vi "Read.vi"(8 "error in (no error)":errorcluster, 11 "I32 Array in":refnum<class "I32 Array.lvclass">) -> (0 "error out":errorcluster, 2 "I32 Array":i32[](array[numeric]), 3 "I32 Array out":refnum<class "I32 Array.lvclass">)   [LabVIEW 2020, in "Data.lvlib" / "I32 Array.lvclass"]
doc: "Read I32 Array."
uses:
  I32 Array.lvclass
  I32 Array.lvclass/I32 Array.ctl
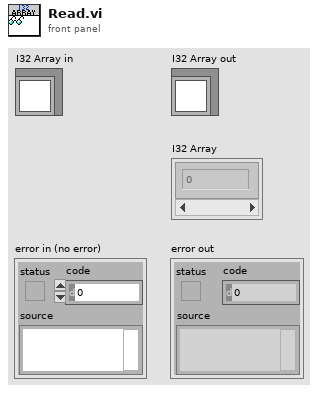
[diagram p1: front panel]
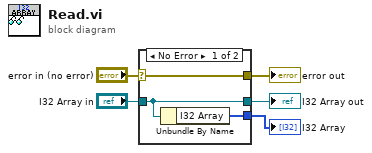
[diagram p0: block diagram]
diagram:
  n1 = case shown="No Error" "error in (no error)" {
    selector: "error in (no error)" -> [w8 w9]
    tunnel: [w8 w9] -> w4
    tunnel: [w7 w10] -> w2
    tunnel: "I32 Array in" -> [w7 w10]
    tunnel: [w6 _] -> w1
    frame No Error {
      n2 = Unbundle By Name(w7) -> ("I32 Array"=w6:i32[])
    }
    frame Error {
    }
  }
  "error out" <- w4
  "I32 Array out" <- w2
  "I32 Array" <- w1
